vi "Terminate.vi"(8 "error in (no error)":errorcluster, 11 "WAMP Client in":refnum<class "WAMP Client.lvclass">) -> (0 "error out":errorcluster, 3 "WAMP Client out":refnum<class "WAMP Client.lvclass">)   [LabVIEW 2020, in "wamplv.lvlib" / "WAMP Client.lvclass"]
uses:
  WAMP Client.lvclass
  TypeDef/Internal Daemon Termination Loop Msg.ctl
  Private/Comm Handlers/ICommHandler/ICommHandler.lvclass
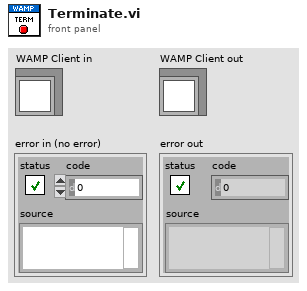
[diagram p1: front panel]
types:
  T1 = typedef "wamplv.lvlib/WAMP Client.lvclass/Termination Reason.ctl" = cluster{"Reason":T2, "Reason URI":string, "Message":string}
  T2 = typedef "wamplv.lvlib/WAMP Client.lvclass/Termination Reason Enum.ctl" = enum16{"Goodbye Received", "Abort Received", "Send Goodbye", "Send Abort", "Read Loop Failure", "Write Loop Failure", "Message Loop Failure"}
  T3 = typedef "wamplv.lvlib/WAMP Client.lvclass/Internal Daemon Termination Loop Msg.ctl" = enum16{"Send Goodbye and Wait For Response", "Send Goodbye and Terminate", "Wait for Goodbye", "Send Abort", "Terminate"}
  T4 = typedef "wamplv.lvlib/WAMP Client.lvclass/WAMP Message Codes.ctl" = u16
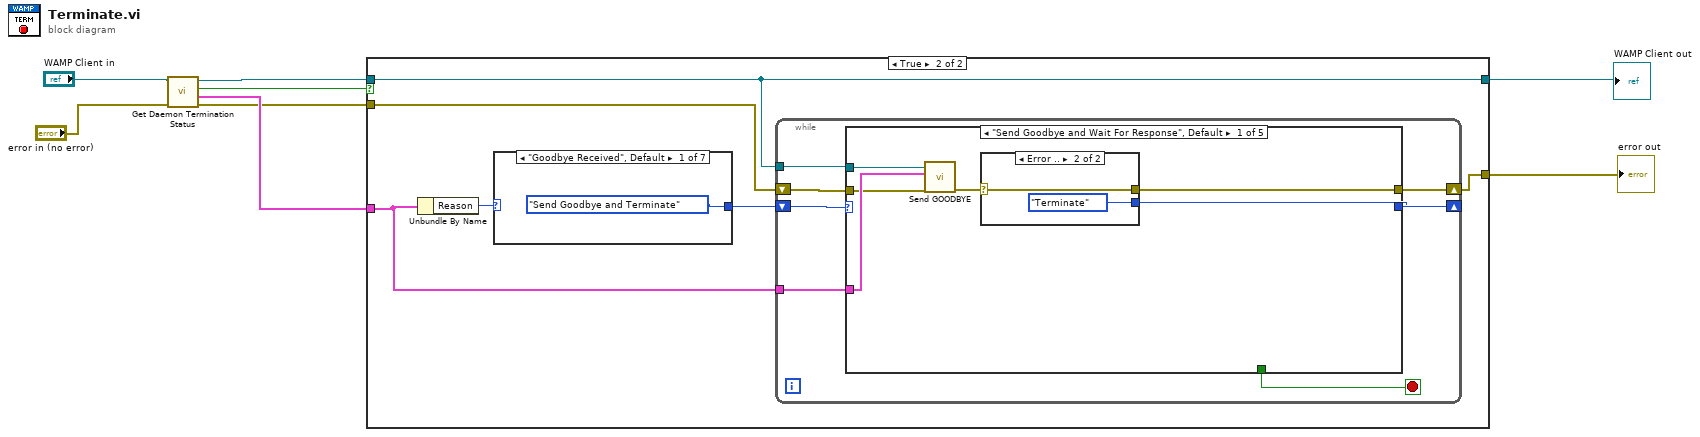
[diagram p0: block diagram]
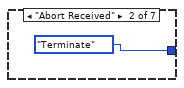
[diagram p3: hidden frame]
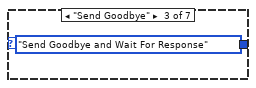
[diagram p4: hidden frame]
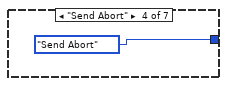
[diagram p5: hidden frame]
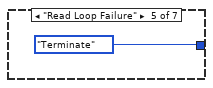
[diagram p6: hidden frame]
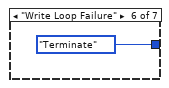
[diagram p7: hidden frame]
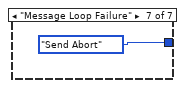
[diagram p8: hidden frame]
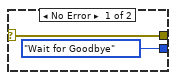
[diagram p9: hidden frame]
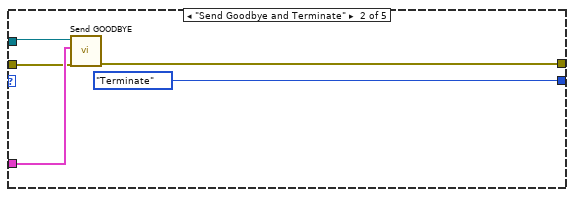
[diagram p10: hidden frame]
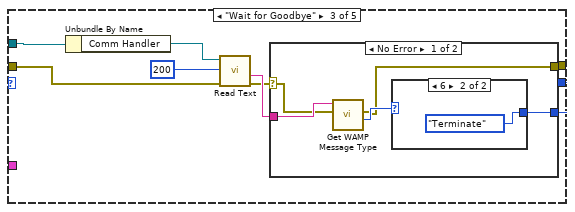
[diagram p11: hidden frame]
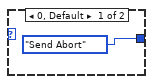
[diagram p12: hidden frame]
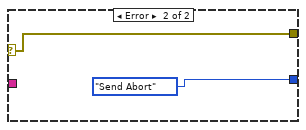
[diagram p13: hidden frame]
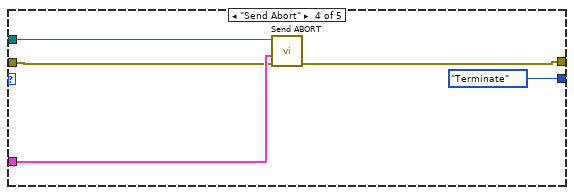
[diagram p14: hidden frame]
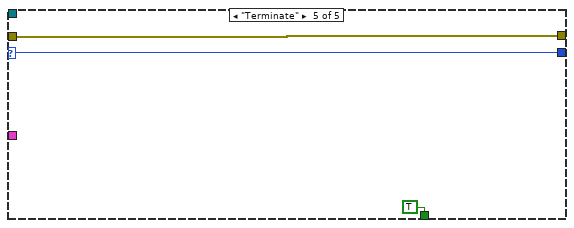
[diagram p15: hidden frame]
diagram:
  n1 = call "Get Daemon Termination Status.vi"("error in (no error)"="error in (no error)", "WAMP Client in"="WAMP Client in") -> ("error out"=w2:errorcluster, "Termination Reason"=w5:T1, "Terminate?"=w3:bool, "WAMP Client out"=w7:refnum<class "WAMP Client.lvclass">)  [unwired: 6 in]
  n2 = case shown="True" w3 {
    tunnel: w7 -> [w9 w11]
    tunnel: w5 -> [_ w14]
    tunnel: [w10 w13] -> w4
    tunnel: w2 -> [w10 w12]
    tunnel: [w9 w11] -> w1
    frame False {
    }
    frame True {
      n3 = Unbundle By Name(w14) -> ("Reason"=w15:T2)
      n4 = case shown="\"Goodbye Received\", Default" w15 {
        tunnel: [Internal_Daemon_Termination_Loop_Msg."Send Goodbye and Terminate" ("Termination Loop Msg") Internal_Daemon_Termination_Loop_Msg."Terminate" ("Termination Loop Msg") Internal_Daemon_Termination_Loop_Msg."Send Goodbye and Wait For Response" ("Termination Loop Msg") Internal_Daemon_Termination_Loop_Msg."Send Abort" ("Termination Loop Msg") Internal_Daemon_Termination_Loop_Msg."Terminate" ("Termination Loop Msg") Internal_Daemon_Termination_Loop_Msg."Terminate" ("Termination Loop Msg") Internal_Daemon_Termination_Loop_Msg."Send Abort" ("Termination Loop Msg")] -> w16
        frame "Goodbye Received", Default {
        }
        frame "Abort Received" {
        }
        frame "Send Goodbye" {
        }
        frame "Send Abort" {
        }
        frame "Read Loop Failure" {
        }
        frame "Write Loop Failure" {
        }
        frame "Message Loop Failure" {
        }
      }
      n5 = while {
        shift-right: [w27] -> _
        shift-left: w16 -> [w30]
        tunnel: w11 -> [w29]
        tunnel: w14 -> [w28]
        shift-right: [w25] -> w13
        shift-left: w12 -> [w24]
        stop <- w26 stop-if-true
        n6 = case shown="\"Send Goodbye and Wait For Response\", Default" w30 {
          selector: w30 -> [_ _ _ _ w69]
          tunnel: w29 -> [w34 w45 w53 w67 _]
          tunnel: w28 -> [w33 w43 _ w65 _]
          tunnel: [w36 Internal_Daemon_Termination_Loop_Msg."Terminate" ("Termination Loop Msg") w50 Internal_Daemon_Termination_Loop_Msg."Terminate" ("Termination Loop Msg") w69] -> w27
          tunnel: [_ _ _ _ TRUE] -> w26
          tunnel: [w35 w42 w49 w63 w68] -> w25
          tunnel: w24 -> [w32 w41 w47 w64 w68]
          frame "Send Goodbye and Wait For Response", Default {
            n7 = call-dynamic "Send GOODBYE.vi"("error in (no error)"=w32, "Termination Reason"=w33, "WAMP Client in"=w34) -> ("error out"=w31:errorcluster)  [unwired: 7 in, 1 out]
            n8 = case shown="Error .." w31 {
              selector: w31 -> [w37 w39]
              tunnel: [Internal_Daemon_Termination_Loop_Msg."Wait for Goodbye" ("Termination Loop Msg") Internal_Daemon_Termination_Loop_Msg."Terminate" ("Termination Loop Msg")] -> w36
              tunnel: [w37 w39] -> w35
              frame No Error {
              }
              frame Error {
              }
            }
          }
          frame "Send Goodbye and Terminate" {
            n9 = call-dynamic "Send GOODBYE.vi"("error in (no error)"=w41, "Termination Reason"=w43, "WAMP Client in"=w45) -> ("error out"=w42:errorcluster)  [unwired: 7 in, 1 out]
          }
          frame "Wait for Goodbye" {
            n10 = Unbundle By Name(w53) -> ("Comm Handler"=w52:refnum<class "ICommHandler.lvclass">)
            n11 = call-dynamic "Read Text.vi"("error in (no error)"=w47, "timeout ms (5000)"=200, "ICommHandler in"=w52) -> ("error out"=w46:errorcluster, "String"=w51:string)  [unwired: 4 in, 1 out]
            n12 = case shown="No Error" w46 {
              selector: w46 -> [w55 w61]
              tunnel: w51 -> [w58 _]
              tunnel: [w56 Internal_Daemon_Termination_Loop_Msg."Send Abort" ("Termination Loop Msg")] -> w50
              tunnel: [w54 w61] -> w49
              frame No Error {
                n13 = call "Get WAMP Message Type.vi"("error in (no error)"=w55, "JSON"=w58) -> ("Message Codes"=w57:T4, "error out"=w54:errorcluster)  [unwired: 6 in, 2 out]
                n14 = case shown="6" w57 {
                  tunnel: [Internal_Daemon_Termination_Loop_Msg."Send Abort" ("Termination Loop Msg") Internal_Daemon_Termination_Loop_Msg."Terminate" ("Termination Loop Msg")] -> w56
                  frame 0, Default {
                  }
                  frame 6 {
                  }
                }
              }
              frame Error {
              }
            }
          }
          frame "Send Abort" {
            n15 = call-dynamic "Send ABORT.vi"("error in (no error)"=w64, "Abort Request"=w65, "WAMP Client in"=w67) -> ("error out"=w63:errorcluster)  [unwired: 7 in, 1 out]
          }
          frame "Terminate" {
          }
        }
      }
    }
  }
  "error out" <- w4
  "WAMP Client out" <- w1
